vi "UnBindControlFrimMatlabValue.vi"(10 "Controls[]":refnum<vi>[](array[refnum]), 11 "Control":refnum<vi>) -> (3 "Bound Events":T1[](array[typedef]))   [LabVIEW 2017]
uses:
  Types/ControlValueChangeEventBindingType.ctl
panel:
  in  "ExpID":string
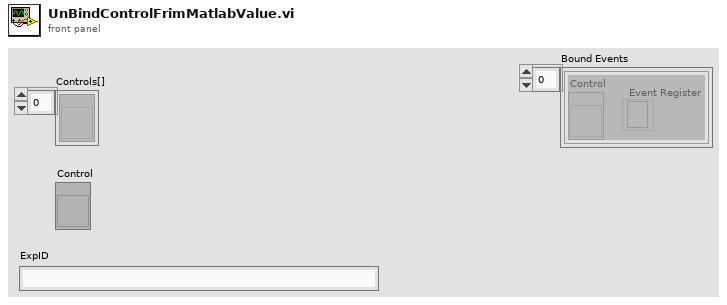
[diagram p1: front panel]
types:
  T1 = typedef "ControlValueChangeEventBindingType.ctl" = cluster{"Control":refnum<vi>, "Event Register":refnum<event-registration>}
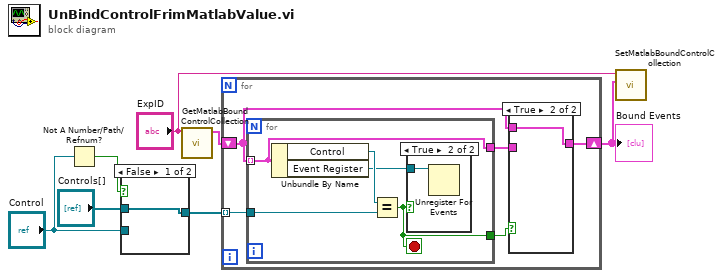
[diagram p0: block diagram]
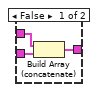
[diagram p2: hidden frame]
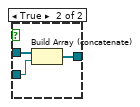
[diagram p4: hidden frame]
diagram:
  n1 = Not A Number/Path/Refnum?(number/path/refnum="Control") -> (NaN/Path/Refnum?=w7:bool)
  n2 = case shown="False" w7 {
    tunnel: "Controls[]" -> [w8 w11]
    tunnel: "Control" -> [_ w10]
    tunnel: [w8 w9] -> w4
    frame False {
    }
    frame True {
      n3 = Build Array (concatenate)(w11, w10) -> (w9:refnum<vi>[])
    }
  }
  n4 = call "GetMatlabBoundControlCollection.vi"("ExpID"="ExpID") -> ("Bound Controls"=w1:T1[])  [unwired: 10 in]
  n5 = for {
    tunnel: w4 -> [w16] mode=indexing
    shift-right: [w12] -> w2
    shift-left: w1 -> [w13]
    n6 = for {
      tunnel: w16 -> [w24]
      tunnel: [w23] -> w15
      tunnel: w13 -> [w21] mode=indexing
      tunnel: [w21] -> w14
      stop <- w23 stop-if-true
      n7 = Unbundle By Name(w21) -> ("Control"=w25:refnum<vi>, "Event Register"=w22:refnum<event-registration>)
      n8 = Equal?(x=w25, y=w24) -> (x = y?=w23:bool)
      n9 = case shown="True" w23 {
        tunnel: w22 -> [_ w26]
        frame False {
        }
        frame True {
          n10 = Unregister For Events(event registration refnum=w26) -> ()  [unwired: 1 in, 1 out]
        }
      }
    }
    n11 = case shown="True" w15 {
      tunnel: w14 -> [w19 _]
      tunnel: w13 -> [w18 w20]
      tunnel: [w17 w20] -> w12
      frame False {
        n12 = Build Array (concatenate)(w18, w19) -> (w17:T1[])
      }
      frame True {
      }
    }
  }
  "Bound Events" <- w2
  n13 = call "SetMatlabBoundControlCollection.vi"("Bound controls"=w2, "ExpID"="ExpID") -> ()  [unwired: 10 in]
